vi "kozv.vi"() -> ()   [LabVIEW 2019]
uses:
  <vilib>/Platform/TimedLoop/XDataNode/timing_clust.ctl
  <vilib>/Platform/TimedLoop/XDataNode/nitl_modes.ctl
  <vilib>/Platform/TimedLoop/XDataNode/wakeup.ctl
  <vilib>/Analysis/baseanly.llb/Mean (DBL).vi
  <vilib>/platform/TimedLoop/XDataNode/XDataNode.xnode
  <vilib>/Platform/TimedLoop/XDataNode/XDNodeRunTimeDep.lvlib
  <vilib>/Analysis/NI_AALBase.lvlib
panel:
  in  "k_loc":dbl
  in  "T_loc":dbl
  in  "Boolean":bool
  out "V":dbl
  out "Vtest":dbl
  out "S":dbl
  out "toado":dbl[][](array[numeric])
  in  "toadothucong":dbl[][](array[numeric])
  in  "phi_end":dbl
  in  "phi_start":dbl
  in  "phi_step":dbl=0.08
  out "Waveform Chart 2":dbl(graph)
  in  "Kps":dbl=7.0
  out "dec time":dbl
  in  "resetgraph2":bool=TRUE caption="Reset"
  out "duty3":dbl
  out "duty2":dbl
  out "duty1":dbl
  in  "Reset":bool
  out "Y_sp":dbl
  out "X_sp":dbl
  out "Y_ph":dbl
  out "X_ph":dbl
  out "Map":cluster{"Y":dbl[], "Y":dbl[]}[](graph)
  out "V3_sp":dbl
  out "V3_ph":dbl
  out "Waveform Chart":T1(graph)
  in  "Kiv":dbl=0.2454
  in  "Kpv":dbl=0.00408
  out "V2_ph":dbl
  out "V1_ph":dbl
  out "V2_sp":dbl
  out "V1_sp":dbl
  in  "Start":bool
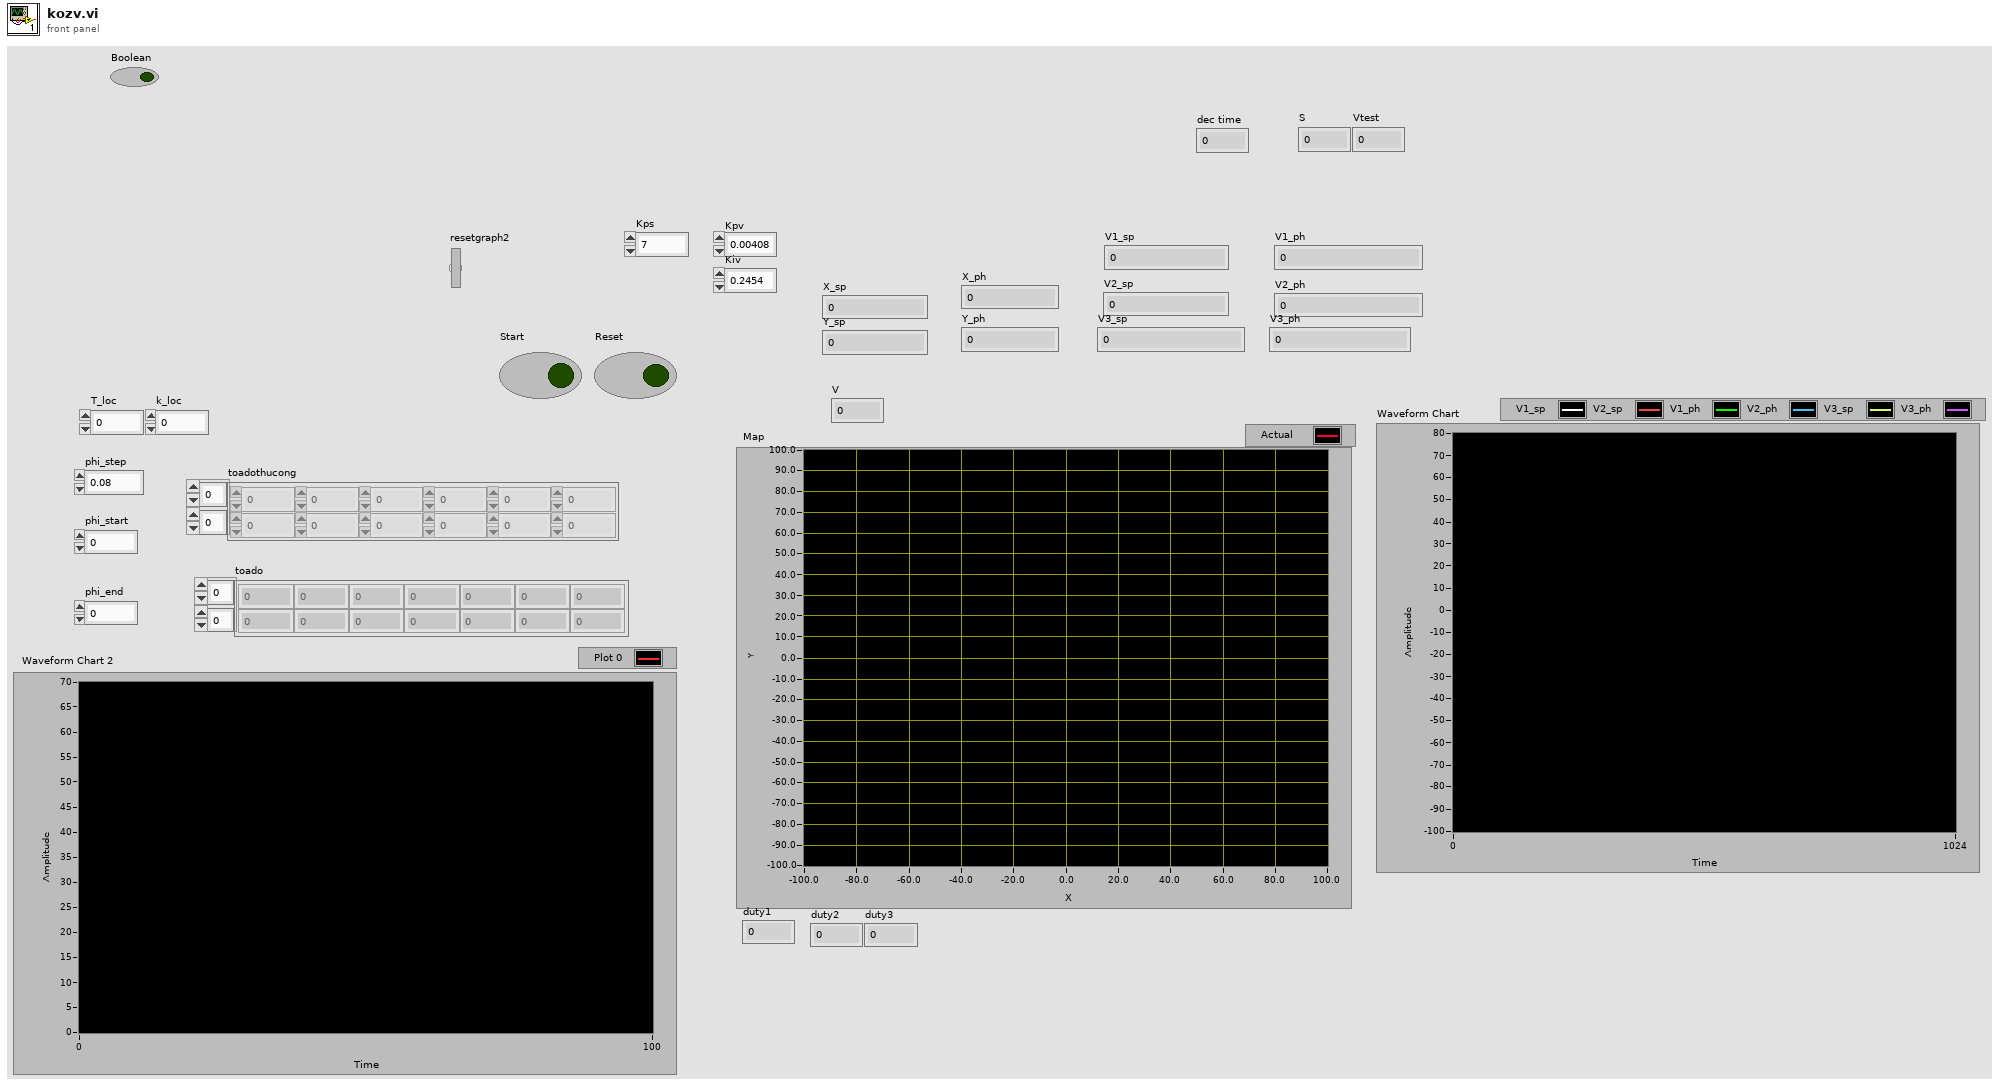
[diagram p1: front panel]
types:
  T1 = cluster{dbl, dbl, "V1_ph":dbl, "V2_ph":dbl, dbl, "V3_ph":dbl}
  T2 = typedef "XDNodeRunTimeDep.lvlib/timing_clust.ctl" = cluster{"Expected End [f-1]":u64, "Actual End [f-1]":u64, "Finished Late? [f-1]":bool, "Expected End [i-1]":u64, "Actual End [i-1]":u64, "Finished Late? [i-1]":bool, "Expected Start [i]":u64, "Actual Start [i]":u64, "Expected Start [f]":u64, "Actual Start [f]":u64, "Source Name":string, "Structure Name":string, "Period":i64, "Deadline":i64, "Offset":i64, "Start":i64, "Priority":i32, "Timeout":i32, "Mode":T3, "Wakeup Reason":T4, "Error":errorcluster, "Source Type":string, "Secondary Source Type":string, "Global End Time":u64, "Global Start Time":u64, "Frame Duration":u64, "Iteration Duration":u64, "Assigned CPU":i32, "I/O Scan Engine Mode":u32}
  T3 = typedef "XDNodeRunTimeDep.lvlib/nitl_modes.ctl" = enum32{"No Change", "Process missed periods, maintain original phase", "Discard missed periods, maintain original phase", "Process missed periods, ignore original phase", "Discard missed periods, ignore original phase"}
  T4 = typedef "XDNodeRunTimeDep.lvlib/wakeup.ctl" = enum32{"Normal", "Aborted", "Asynchronous wakeup", "Timing source error", "Timed loop error", "Timeout"}
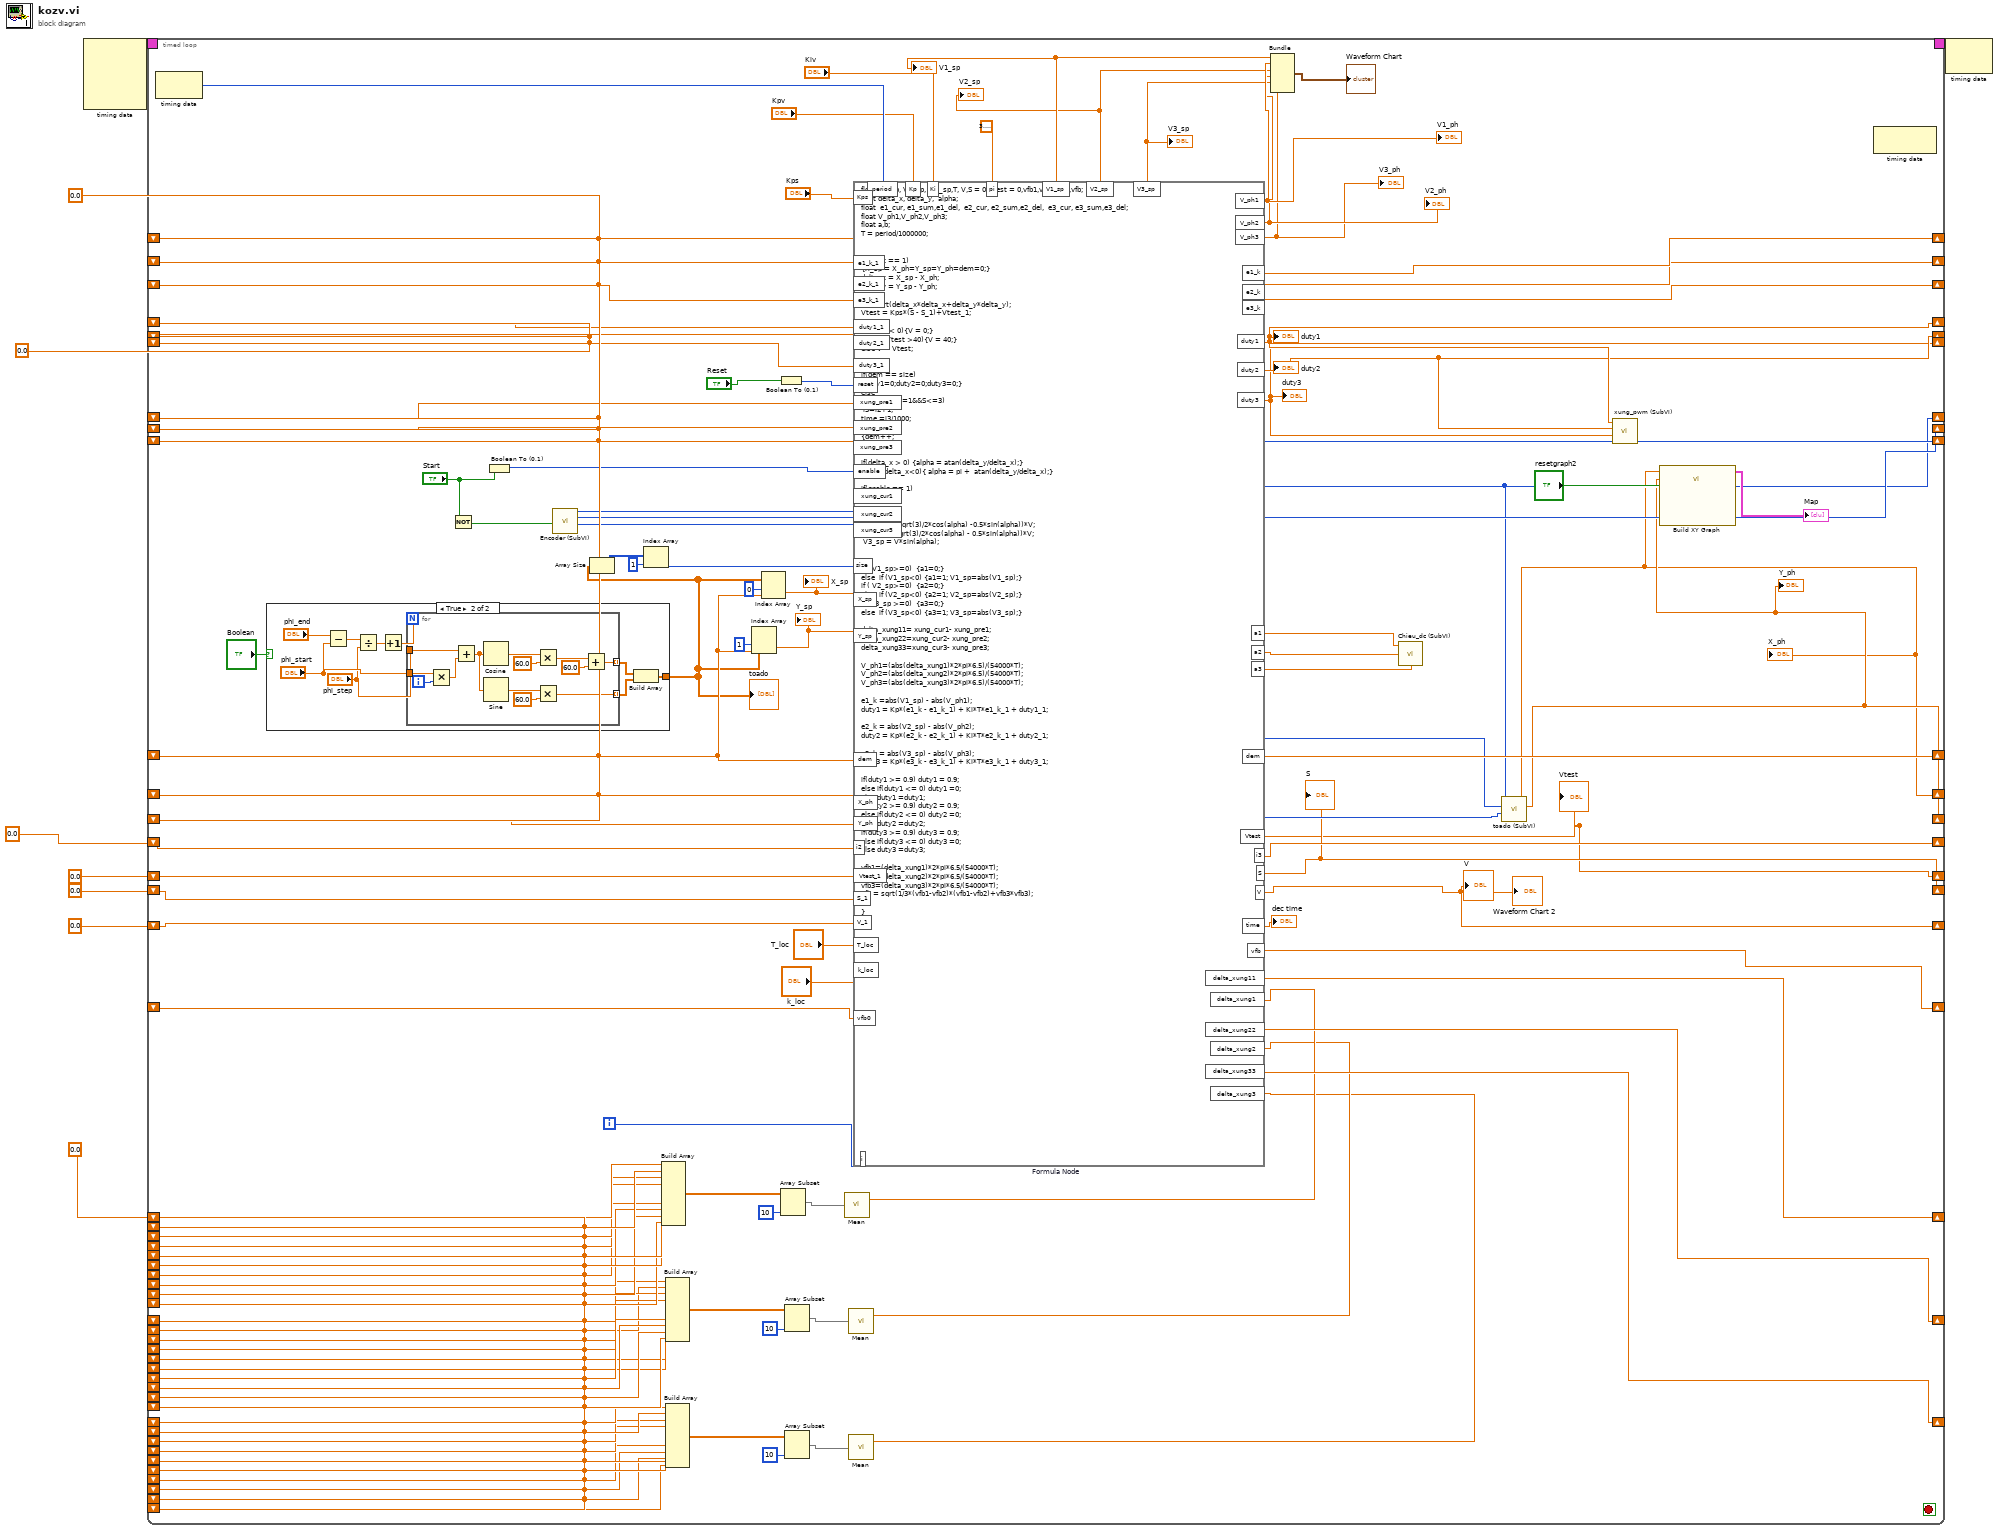
[diagram p0: block diagram]
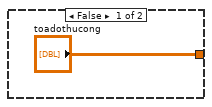
[diagram p2: hidden frame]
diagram:
  w5 = 0.0 ("delta_xung11")
  w4 = 0.0 ("duty1")
  w7 = 0.0 ("e1")
  n1 = node-c288() -> (w9:T2)  [unwired: 4 in]
  n2 = timed-loop {
    timing: w9 -> [_]
    timing-out: [_] -> w8
    shift-right: [w123] -> _
    shift-left: w7 -> [w121]
    shift-right: [w122] -> _
    shift-left: w7 -> [w120]
    shift-right: [w25] -> _
    shift-left: w7 -> [w109]
    shift-right: [w84] -> _
    shift-left: w7 -> [w117]
    shift-right: [w112] -> _
    shift-left: w7 -> [w111]
    shift-right: [w83] -> _
    shift-left: w7 -> [w110]
    shift-right: [w26] -> _
    shift-left: w7 -> [w108]
    shift-right: [w82] -> _
    shift-left: w7 -> [w107]
    shift-right: [w106] -> _
    shift-left: w7 -> [w22]
    shift-right: [w86] -> _
    shift-left: _ -> [w88]
    shift-right: [w81] -> _
    shift-left: 0.0 ("i3") -> [w23]
    shift-right: [w79] -> _
    shift-left: w4 -> [w76]
    shift-right: [w78] -> _
    shift-left: w4 -> [w75]
    shift-right: [w77] -> _
    shift-left: w4 -> [w74]
    shift-right: [w32] -> _
    shift-left: w5 -> [w68]
    shift-left: w5 -> [w67]
    shift-left: w5 -> [w66]
    shift-left: w5 -> [w65]
    shift-left: w5 -> [w64]
    shift-left: w5 -> [w63]
    shift-left: w5 -> [w62]
    shift-left: w5 -> [w61]
    shift-left: w5 -> [w60]
    shift-left: w5 -> [w59]
    shift-right: [w31] -> _
    shift-left: w5 -> [w49]
    shift-left: w5 -> [w50]
    shift-left: w5 -> [w51]
    shift-left: w5 -> [w52]
    shift-left: w5 -> [w53]
    shift-left: w5 -> [w54]
    shift-left: w5 -> [w55]
    shift-left: w5 -> [w56]
    shift-left: w5 -> [w57]
    shift-left: w5 -> [w58]
    shift-right: [w30] -> _
    shift-left: w5 -> [w42]
    shift-left: w5 -> [w41]
    shift-left: w5 -> [w40]
    shift-left: w5 -> [w39]
    shift-left: w5 -> [w38]
    shift-left: w5 -> [w37]
    shift-left: w5 -> [w36]
    shift-left: w5 -> [w35]
    shift-left: w5 -> [w34]
    shift-left: w5 -> [w33]
    shift-right: [w14] -> _
    shift-left: 0.0 -> [w18]
    shift-right: [w16] -> _
    shift-left: 0.0 -> [w17]
    shift-right: [w12] -> _
    shift-left: 0.0 -> [w13]
    i -> [w87]
    stop <- _ stop-if-true
    n3 = node-c288() -> (w116:i64)  [unwired: 1 in]
    n4 = case shown="True" "Boolean" {
      tunnel: ["toadothucong" w125] -> w19
      frame False {
      }
      frame True {
        n5 = Subtract(x="phi_end", y="phi_start") -> (x-y=w132:dbl)
        n6 = Divide(x=w132, y="phi_step") -> (x/y=w133:dbl)
        n7 = Increment(x=w133) -> (x+1=w130:dbl)
        n8 = for {
          N: w130 -> [_]
          tunnel: "phi_start" -> [w146]
          tunnel: "phi_step" -> [w145]
          tunnel: [w134] -> w126 mode=indexing
          tunnel: [w138] -> w127 mode=indexing
          i -> [w144]
          n9 = Multiply(x=w145, y=w144) -> (x*y=w143:dbl)
          n10 = Add(x=w146, y=w143) -> (x+y=w137:dbl)
          n11 = Cosine(x=w137) -> (cos(x)=w141:dbl)
          n12 = Sine(x=w137) -> (sin(x)=w136:dbl)
          n13 = Multiply(x=w141, y=60.0) -> (x*y=w139:dbl)
          n14 = Multiply(x=w136, y=60.0) -> (x*y=w134:dbl)
          n15 = Add(x=w139, y=60.0) -> (x+y=w138:dbl)
        }
        n16 = Build Array(w127, w126) -> (w125:dbl[][])
      }
    }
    "toado" <- w19
    n17 = Not(x="Start") -> (.not. x?=w89:bool)
    n18 = Boolean To (0,1)(Boolean="Start") -> (0, 1=w119:i16)
    n19 = call "Encoder (SubVI).vi"("Boolean"=w89) -> ("Counter Value3"=w83:i32, "Counter Value 2"=w84:i32, "Counter Value"=w25:i32)  [unwired: 8 in]
    n20 = Array Size(array=w19) -> (size(s)=w102:i32[])
    n21 = Index Array(array=w102, index=1) -> (element=w100:i32)
    n22 = Build Array(w68, w67, w66, w65, w64, w63, w62, w61, w60, w59) -> (w70:dbl[])
    n23 = Build Array(w49, w50, w51, w52, w53, w54, w55, w56, w57, w58) -> (w47:dbl[])
    n24 = Build Array(w42, w41, w40, w39, w38, w37, w36, w35, w34, w33) -> (w44:dbl[])
    n25 = Index Array(array=w19, index (row)=1 ("disabled index (row)"), index (col)=w22) -> (element=w103:dbl)
    "Y_sp" <- w103
    n26 = Index Array(array=w19, index (row)=0 ("disabled index (row)"), index (col)=w22) -> (element=w104:dbl)
    "X_sp" <- w104
    n27 = Boolean To (0,1)(Boolean="Reset") -> (0, 1=w99:i16)
    n28 = Array Subset(array=w70, length=10) -> (w69:dbl[])  [unwired: 1 in]
    n29 = Array Subset(array=w47, length=10) -> (w48:dbl[])  [unwired: 1 in]
    n30 = Array Subset(array=w44, length=10) -> (w43:dbl[])  [unwired: 1 in]
    n31 = call-poly <vilib>:"Mean.vi"("X"=w69) -> ("mean"=w29:dbl)  [unwired: 1 out]
    n32 = call-poly <vilib>:"Mean.vi"("X"=w48) -> ("mean"=w28:dbl)  [unwired: 1 out]
    n33 = call-poly <vilib>:"Mean.vi"("X"=w43) -> ("mean"=w27:dbl)  [unwired: 1 out]
    n34 = formula code="float V1_sp, V2_sp,  V3_sp,T, V,S = 0,Vtest = 0,vfb1,vfb2,vfb3,vfb;\nfloat delta_x, delta_y,  alpha;\nfloat  e1_cur, e1_sum,e1_del,  e2_cur, e2_sum,e2_del,  e3_cur, e3_sum,e3_del;\nfloat V_ph1,V_ph2,V_ph3;\nfloat a,b;\nT = period/1000000;\n\n\nif(reset == 1)\n{X_sp = X_ph=Y_sp=Y_ph=dem=0;}\ndelta_x = X_sp - X_ph;\ndelta_y = Y_sp - Y_ph;\n\nS = sqrt(delta_x*delta_x+delta_y*delta_y); \nVtest = Kps*(S - S_1)+Vtest_1;\n\nif(Vtest < 0){V = 0;}\nelse if (Vtest >40){V = 40;}\nelse V = Vtest;\n\n\nif(dem == size)\n{duty1=0;duty2=0;duty3=0;}\nelse\n{ if(enable==1&&S<=3)\n i3=i2+1;\ntime =i3/1000;\nif(i3>=30)\n{dem++;\ni2=0;i3=0;}\n\nif(delta_x > 0) {alpha = atan(delta_y/delta_x);}\nelse if(delta_x<0){ alpha = pi +  atan(delta_y/delta_x);}\n\nif(enable == 1)\n{\n\n\nV1_sp = (-sqrt(3)/2*cos(alpha) -0.5*sin(alpha))*V;\nV2_sp = (sqrt(3)/2*cos(alpha) - 0.5*sin(alpha))*V;\n V3_sp = V*sin(alpha); \n\n\nif ( V1_sp>=0)  {a1=0;}\nelse  if (V1_sp<0) {a1=1; V1_sp=abs(V1_sp);}\nif ( V2_sp>=0)  {a2=0;}\nelse  if (V2_sp<0) {a2=1; V2_sp=abs(V2_sp);}\nif (V3_sp >=0)  {a3=0;}\nelse  if (V3_sp<0) {a3=1; V3_sp=abs(V3_sp);}\n\ndelta_xung11= xung_cur1- xung_pre1;\ndelta_xung22=xung_cur2- xung_pre2;\ndelta_xung33=xung_cur3- xung_pre3; \n\nV_ph1=(abs(delta_xung1)*2*pi*6.5)/(54000*T);\nV_ph2=(abs(delta_xung2)*2*pi*6.5)/(54000*T);\nV_ph3=(abs(delta_xung3)*2*pi*6.5)/(54000*T);\n\ne1_k =abs(V1_sp) - abs(V_ph1);\nduty1 = Kp*(e1_k - e1_k_1) + Ki*T*e1_k_1 + duty1_1;\n\ne2_k = abs(V2_sp) - abs(V_ph2);\nduty2 = Kp*(e2_k - e2_k_1) + Ki*T*e2_k_1 + duty2_1;\n\ne3_k = abs(V3_sp) - abs(V_ph3);\nduty3 = Kp*(e3_k - e3_k_1) + Ki*T*e3_k_1 + duty3_1;\n\nif(duty1 >= 0.9) duty1 = 0.9;\nelse if(duty1 <= 0) duty1 =0;\nelse duty1 =duty1;\nif(duty2 >= 0.9) duty2 = 0.9;\nelse if(duty2 <= 0) duty2 =0;\nelse duty2 =duty2;\nif(duty3 >= 0.9) duty3 = 0.9;\nelse if(duty3 <= 0) duty3 =0;\nelse duty3 =duty3;\n\nvfb1=(delta_xung1)*2*pi*6.5/(54000*T);\nvfb2=(delta_xung2)*2*pi*6.5/(54000*T);\nvfb3=(delta_xung3)*2*pi*6.5/(54000*T);\nvfb = sqrt(1/3*(vfb1-vfb2)*(vfb1-vfb2)+vfb3*vfb3);\n}\n}"("Kp"="Kpv", "Ki"="Kiv", "pi"=3.141592653589793, "e1_k_1"=w121, "e2_k_1"=w120, "xung_pre1"=w109, "xung_pre2"=w117, "xung_cur1"=w25, "xung_cur2"=w84, "enable"=w119, "period"=w116, "e3_k_1"=w111, "xung_cur3"=w83, "xung_pre3"=w110, "X_ph"=w108, "X_sp"=w104, "Y_sp"=w103, "Y_ph"=w107, "dem"=w22, "size"=w100, "reset"=w99, "i"=w87, "vfb0"=w88, "i2"=w23, "duty1_1"=w76, "duty2_1"=w75, "duty3_1"=w74, "delta_xung1"=w29, "delta_xung2"=w28, "delta_xung3"=w27, "Kps"="Kps", "Vtest_1"=w18, "S_1"=w17, "V_1"=w13, "T_loc"="T_loc", "k_loc"="k_loc") -> ("V1_sp"=w97:dbl, "V_ph1"=w96:dbl, "V_ph2"=w94:dbl, "e1_k"=w123:dbl, "e2_k"=w122:dbl, "V2_sp"=w95:dbl, "duty1"=w79:dbl, "duty2"=w78:dbl, "e3_k"=w112:dbl, "V_ph3"=w93:dbl, "V3_sp"=w92:dbl, "duty3"=w77:dbl, "a1"=w85:dbl, "a2"=w73:dbl, "a3"=w72:dbl, "dem"=w106:dbl, "vfb"=w86:dbl, "i3"=w81:dbl, "time"=→"dec time":dbl, "delta_xung11"=w32:dbl, "delta_xung22"=w31:dbl, "delta_xung33"=w30:dbl, "S"=w16:dbl, "Vtest"=w14:dbl, "V"=w12:dbl)
    "V1_sp" <- w97
    "V2_sp" <- w95
    "V1_ph" <- w96
    "V2_ph" <- w94
    "V3_ph" <- w93
    "V3_sp" <- w92
    "duty1" <- w79
    "duty2" <- w78
    "duty3" <- w77
    "Waveform Chart 2" <- w12
    "S" <- w16
    "Vtest" <- w14
    "V" <- w12
    n35 = Bundle(w97, w96, w95, w94, w92, w93) -> (→"Waveform Chart":cluster{dbl, dbl, dbl, dbl, dbl, dbl})  [unwired: 1 in]
    n36 = call "Chieu_dc (SubVI).vi"("a3"=w72, "a2"=w73, "a1"=w85) -> ()
    n37 = call "toado (SubVI).vi"("X3"=w83, "X2"=w84, "X1"=w25) -> ("Y_ph"=w82:dbl, "X_ph"=w26:dbl)  [unwired: 7 in]
    "X_ph" <- w26
    "Y_ph" <- w82
    n38 = call "xung_pwm (SubVI).vi"("duty3 in"=w77, "duty2 in"=w78, "duty1 in"=w79) -> ()  [unwired: 6 in, 3 out]
    n39 = call "Build XY Graph"("Reset"="resetgraph2", "Y Input"=w82, "X Input"=w26) -> ("XY Graph"=→"Map":cluster{"X":dbl[], "Y":dbl[]}[])  [unwired: 7 in, 1 out]
    n40 = node-c288() -> ()  [unwired: 1 in, 1 out]
  }
  n41 = node-c288(w8) -> ()  [unwired: 1 out]
